vi "dfd_Dummy_INT Filtering wStateAB.vi"(8 "stateB in":i32[](array[numeric]), 9 "stateA in":i32[](array[numeric]), 11 "x":i16) -> (0 "stateB out":i32[](array[numeric]), 1 "stateA out":i32[](array[numeric]), 3 "y":i16)   [LabVIEW 2017]
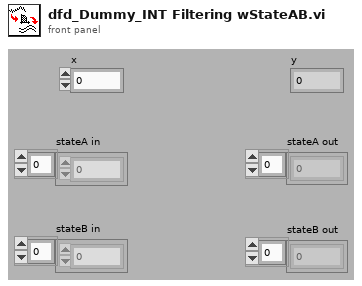
[diagram p1: front panel]
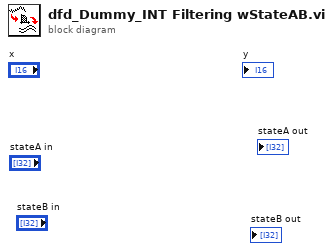
[diagram p0: block diagram]
diagram:
